vi "Set Key Persistence.vi"(4 "Return matching names? [F]":bool, 5 "Key name":string, 6 "Persistent? [F]":bool, 7 "Section name":string, 8 "error in (no error)":errorcluster, 9 "Use Key Regex? [F]":bool, 10 "Use Section Regex? [F]":bool, 11 "Carya Config in":refnum<class "Carya Config.lvclass">) -> (0 "error out":errorcluster, 1 "Key names":string[](array[string]), 2 "Section names":string[](array[string]), 3 "Carya Config out":refnum<class "Carya Config.lvclass">)   [LabVIEW 2013, in "Carya Config.lvclass"]
doc: "Copyright 2018, Carya Automatisering, Wiebe Walstra."
uses:
  Carya Config.lvclass
  CConfig Object/Data.ctl
  CConfig Object/Add Results Query/Add Results Query.lvclass
  CConfig Object/Step In Query/Step In Query.lvclass
  CConfig Object/Composite Query/Composite Query.lvclass
  CConfig Object/Loop Query/Match Query/Match Query.lvclass
  CConfig Object/Set Query/Set Query.lvclass
  CConfig Object/CConfig Object.lvclass
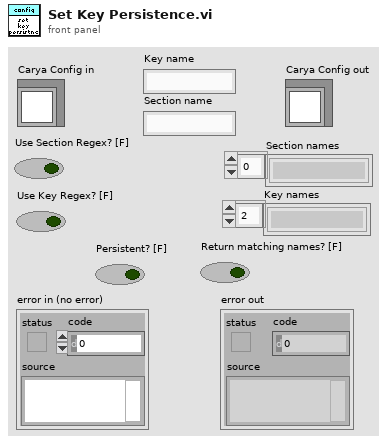
[diagram p1: front panel]
types:
  T1 = typedef "CConfig Object.lvclass/Data.ctl" = enum16{"pre", "name", "middle", "value", "post", "newline", "persistant", "tagged", "type"}
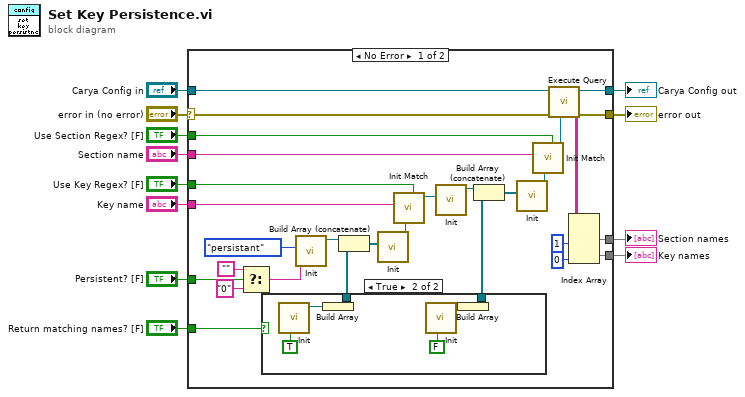
[diagram p0: block diagram]
diagram:
  n1 = case shown="No Error" "error in (no error)" {
    selector: "error in (no error)" -> [w27 w49]
    tunnel: [w26 w49] -> w11
    tunnel: [w25 w48] -> w9
    tunnel: "Carya Config in" -> [w24 w48]
    tunnel: "Section name" -> [w41 _]
    tunnel: "Key name" -> [w40 _]
    tunnel: "Use Section Regex? [F]" -> [w22 _]
    tunnel: "Use Key Regex? [F]" -> [w23 _]
    tunnel: [w39 _] -> w4
    tunnel: [w38 _] -> w3
    tunnel: "Return matching names? [F]" -> [w19 _]
    tunnel: "Persistent? [F]" -> [w17 _]
    frame No Error {
      n2 = Select(t="", s=w17, f="0") -> (s? t:f=w13:string)
      n3 = case shown="True" w19 {
        tunnel: [_ w43] -> w33
        tunnel: [_ w42] -> w32
        frame False {
        }
        frame True {
          n4 = call "Init.vi"("Concatenate\\Build [T, Concatenate]"=TRUE ("Concatenate\\Build [T, Concatenate]")) -> ("Find First Query out"=w46:refnum<class "Add Results Query.lvclass">)  [unwired: 9 in, 1 out]
          n5 = Build Array(w46) -> (w43:refnum<class "Add Results Query.lvclass">[])
          n6 = call "Init.vi"("Concatenate\\Build [T, Concatenate]"=FALSE ("Concatenate\\Build [T, Concatenate]")) -> ("Find First Query out"=w45:refnum<class "Add Results Query.lvclass">)  [unwired: 9 in, 1 out]
          n7 = Build Array(w45) -> (w42:refnum<class "Add Results Query.lvclass">[])
        }
      }
      n8 = call "Init.vi"("Value"=w13, "Data [value]"=Data."persistant") -> ("Set Query out"=w18:refnum<class "Set Query.lvclass">)  [unwired: 8 in, 1 out]
      n9 = Build Array (concatenate)(w18, w33) -> (w34:refnum<class "CConfig Query.lvclass">[])
      n10 = call "Init.vi"("Queries"=w34) -> ("Step In Query out"=w35:refnum<class "CConfig Query.lvclass">)  [unwired: 9 in, 1 out]
      n11 = call "Init Match.vi"("Regex [F]"=w23, "Found"=w35, "Data"=w40) -> ("Find First Query out"=w20:refnum<class "Loop Query.lvclass">)  [unwired: 7 in, 1 out]
      n12 = call "Init.vi"("Config Query"=w20) -> ("Step In Query out"=w29:refnum<class "Step In Query.lvclass">)  [unwired: 9 in, 1 out]
      n13 = Build Array (concatenate)(w29, w32) -> (w28:refnum<class "CConfig Query.lvclass">[])
      n14 = call "Init.vi"("Queries"=w28) -> ("Step In Query out"=w30:refnum<class "CConfig Query.lvclass">)  [unwired: 9 in, 1 out]
      n15 = call "Init Match.vi"("Regex [F]"=w22, "Found"=w30, "Data"=w41) -> ("Find First Query out"=w21:refnum<class "Loop Query.lvclass">)  [unwired: 7 in, 1 out]
      n16 = call-dynamic "Execute Query.vi"("Config Query in"=w21, "error in (no error)"=w27, "Carya Config in"=w24) -> ("error out"=w26:errorcluster, "Results"=w36:string[][], "Carya Config out"=w25:refnum<class "Carya Config.lvclass">)  [unwired: 4 in, 2 out]
      n17 = Index Array(array=w36, index (col) #1=1 ("disabled index (col)"), index (col) #2=0 ("index (col)")) -> (element #1=w39:string[], element #2=w38:string[])  [unwired: 2 in]
    }
    frame Error {
    }
  }
  "error out" <- w11
  "Carya Config out" <- w9
  "Key names" <- w3
  "Section names" <- w4
